vi "entryDFSM_Busy.vi"(0 "NInstrSim":refnum<class "NInstrSim.lvclass">, 3 "DFSM Internal in":T1, 5 "error in (no error)":errorcluster) -> (14 "dup NInstrSim":refnum<class "NInstrSim.lvclass">, 17 "DFSM Internal out":T1, 19 "error out":errorcluster)   [LabVIEW 2009, in "HB_Device_Examples.lvlib" / "NInstrSim.lvclass"]
doc: "This VI performs <B>entry</B> action of DeviceFSM.Busy.\n\n<b>Hint:</b> This is a dynamic dispatch VI to be implemented by child classes."
uses:
  NInstrSim.lvclass
  lib.lib/HGF_LVC/HGF_StateCharts/HGF_DeviceFSM/HGF_DeviceFSM_Internals.ctl
  lib.lib/HGF_LVC/HGF_DeviceBaseClasses/HGF_VISADevice/HGF_VISADevice.lvclass
  lib.lib/HGF_LVC/HGF_DeviceBaseClasses/HGF_DeviceBaseClasses.lvlib
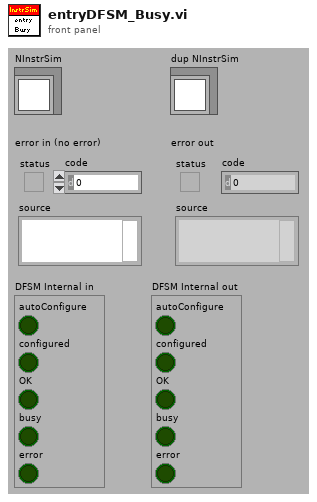
[diagram p1: front panel]
types:
  T1 = typedef "HGF_DeviceBaseClasses.lvlib/HGF_DeviceFSM_Internals.ctl" = cluster{"autoConfigure":bool, "configured":bool, "OK":bool, "busy":bool, "error":bool}
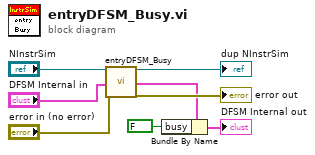
[diagram p0: block diagram]
diagram:
  n1 = call-parent "entryDFSM_Busy.vi"("HGF_DeviceBase"="NInstrSim", "DFSM Internal in"="DFSM Internal in", "error in (no error)"="error in (no error)") -> ("dup HGF_DeviceBase"=→"dup NInstrSim":refnum<class "NInstrSim.lvclass">, "DFSM Internal out"=w4:T1, "error out"=→"error out":errorcluster)  [unwired: 14 out]
  n2 = Bundle By Name(cluster=w4, "busy"=FALSE) -> (→"DFSM Internal out":T1)
